vi "Excel Table.vi"(6 "name":string, 8 "error in (no error)":errorcluster, 9 "table":string[][](table), 10 "start (0, 0)":cluster{"row":i32, "column":i32}, 11 "report in":refnum<class "NI_report.lvclass">) -> (0 "error out":errorcluster, 3 "report out":refnum<class "NI_report.lvclass">)   [LabVIEW 2020, in "varilib.lvlib"]
doc: "Inserts a table into a Microsoft Excel report. Do not change the format of cells."
uses:
  varilib.lvlib
  <vilib>/addons/_office/NI_ReportGenerationToolkit.lvlib
  <vilib>/Utility/NIReport.llb/Excel/NI_Excel.lvclass
  <vilib>/Utility/NIReport.llb/NI_report.lvclass
panel:
  in  "column width (1)":dbl=-1.0 format="%0.2f"
  in  "measurement system":u16(ring) caption="measurement system\nfor column width (US)" items=["US", "Metric"]
  out "Row":i32
  out "Column":i32
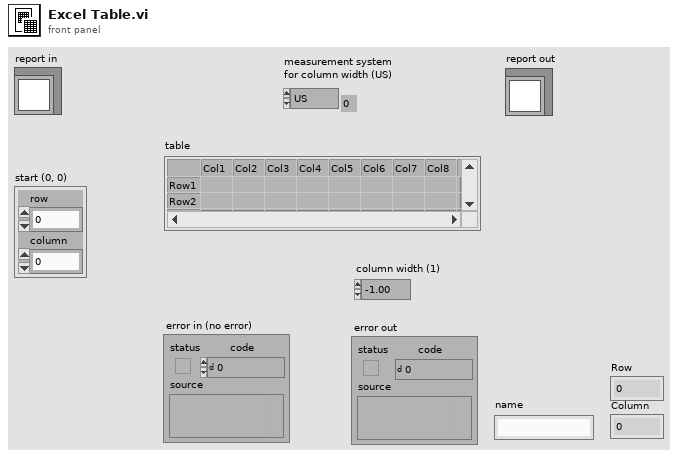
[diagram p1: front panel]
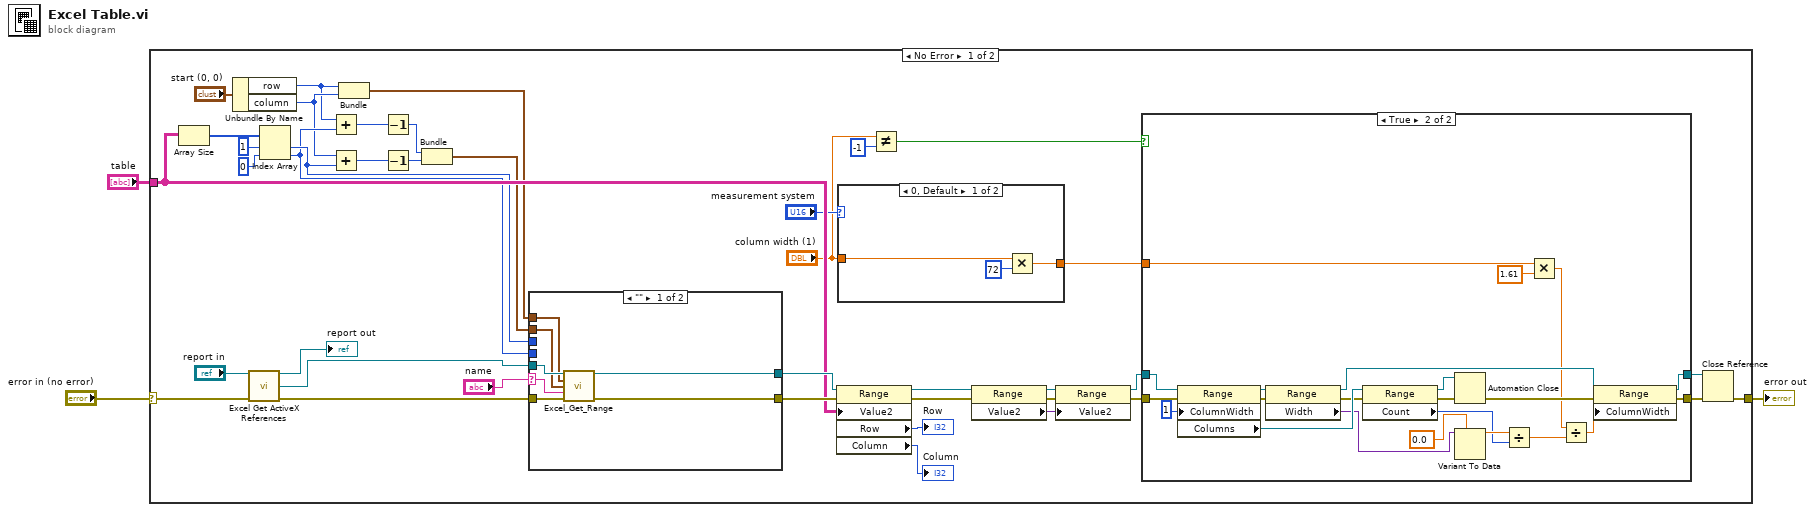
[diagram p0: block diagram]
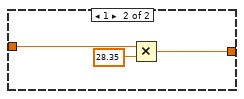
[diagram p2: hidden frame]
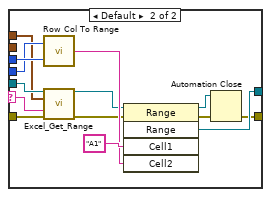
[diagram p4: hidden frame]
diagram:
  n1 = case shown="No Error" "error in (no error)" {
    selector: "error in (no error)" -> [w21 w95]
    tunnel: "table" -> [w39 _]
    tunnel: [w35 w95] -> w2
    frame No Error {
      n2 = Array Size(array=w39) -> (size(s)=w42:i32[])
      n3 = Unbundle By Name("start (0, 0)") -> ("row"=w4:i32, "column"=w5:i32)
      n4 = call <vilib>:"Excel Get ActiveX References.vi"("report in"="report in", "error in (no error)"=w21) -> ("report out"=→"report out":refnum<class "NI_report.lvclass">, "Excel._Worksheet"=w17:refnum<k7>, "error out"=w20:errorcluster)  [unwired: 7 in, 4 out]
      n5 = Index Array(array=w42, index #1=1, index #2=0) -> (element #1=w38:i32, element #2=w23:i32)
      n6 = Add(x=w4, y=w23) -> (x+y=w29:i32)
      n7 = Add(x=w5, y=w38) -> (x+y=w28:i32)
      n8 = Bundle("row"=w4, "column"=w5) -> (w30:cluster{"row":i32, "column":i32})  [unwired: 1 out]
      n9 = Decrement(x=w29) -> (x-1=w26:i32)
      n10 = Decrement(x=w28) -> (x-1=w25:i32)
      n11 = Bundle(w26, w25) -> (w27:cluster{i32, i32})  [unwired: 1 out]
      n12 = case shown="\"\"" "name" {
        selector: "name" -> [w74 w82]
        tunnel: [w80 w94] -> w41
        tunnel: [w79 w88] -> w40
        tunnel: w17 -> [w78 w85]
        tunnel: w20 -> [w77 w84]
        tunnel: w23 -> [_ w90]
        tunnel: w38 -> [_ w91]
        tunnel: w30 -> [w76 w83]
        tunnel: w27 -> [w75 _]
        frame "" {
          n13 = call <vilib>:"Excel_Get_Range.vi"("Excel._Worksheet"=w78, "start"=w76, "end"=w75, "name"=w74, "error in (no error)"=w77) -> ("Range"=w80:refnum<k7>, "error out"=w79:errorcluster)  [unwired: 1 in, 8 out]
        }
        frame Default {
          n14 = call <vilib>:"Row Col To Range.vi"("Column"=w91, "Row"=w90) -> ("Output String"=w92:string)
          n15 = call <vilib>:"Excel_Get_Range.vi"("Excel._Worksheet"=w85, "start"=w83, "name"=w82, "error in (no error)"=w84) -> ("Range"=w81:refnum<k7>, "error out"=w86:errorcluster)  [unwired: 1 in, 9 out]
          n16 = invoke class="Range" method="Range"(reference=w81, error in=w86, "Cell1"="A1", "Cell2"=w92) -> (reference out=w87:refnum<k7>, error out=w89:errorcluster, "Range"=w94:refnum<k7>)  [unwired: 1 in, 2 out]
          n17 = Automation Close(3:w89, 5:w87) -> (0:w88:errorcluster)
        }
      }
      n18 = property class="Range"(reference=w41, error in=w40, "Value2"=w39) -> (reference out=w32:refnum<k7>, error out=w31:errorcluster, "Row"=→"Row":i32, "Column"=→"Column":i32)
      n19 = case shown="0, Default" "measurement system" {
        tunnel: "column width (1)" -> [w46 w48]
        tunnel: [w45 w47] -> w13
        frame 0, Default {
          n20 = Multiply(x=w46, y=72) -> (x*y=w45:dbl)
        }
        frame 1 {
          n21 = Multiply(x=w48, y=28.35) -> (x*y=w47:dbl)
        }
      }
      n22 = Not Equal?(x="column width (1)", y=-1) -> (x != y?=w15:bool)
      n23 = property class="Range"(reference=w32, error in=w31) -> (reference out=w11:refnum<k7>, error out=w10:errorcluster, "Value2"=w7:variant)
      n24 = property class="Range"(reference=w11, error in=w10, "Value2"=w7) -> (reference out=w9:refnum<k7>, error out=w8:errorcluster)
      n25 = case shown="True" w15 {
        tunnel: w9 -> [w51 w73]
        tunnel: w8 -> [w50 w72]
        tunnel: [w50 w70] -> w36
        tunnel: [w51 w71] -> w37
        tunnel: w13 -> [_ w52]
        frame False {
        }
        frame True {
          n26 = property class="Range"(reference=w73, error in=w72, "ColumnWidth"=1) -> (reference out=w59:refnum<k7>, error out=w57:errorcluster, "Columns"=w68:refnum<k7>)
          n27 = property class="Range"(reference=w59, error in=w57) -> (reference out=w58:refnum<k7>, error out=w56:errorcluster, "Width"=w55:variant)
          n28 = property class="Range"(reference=w68, error in=w56) -> (reference out=w64:refnum<k7>, error out=w63:errorcluster, "Count"=w66:i32)
          n29 = Automation Close(3:w63, 5:w64) -> (0:w62:errorcluster)
          n30 = Variant To Data(type=0.0, Variant=w55) -> (data=w67:dbl)  [unwired: 1 in, 1 out]
          n31 = Divide(x=w67, y=w66) -> (x/y=w65:dbl)
          n32 = Multiply(x=w52, y=1.61) -> (x*y=w54:dbl)
          n33 = Divide(x=w54, y=w65) -> (x/y=w61:dbl)
          n34 = property class="Range"(reference=w58, error in=w62, "ColumnWidth"=w61) -> (reference out=w71:refnum<k7>, error out=w70:errorcluster)
        }
      }
      n35 = Close Reference(reference=w37, error in (no error)=w36) -> (error out=w35:errorcluster)
    }
    frame Error {
    }
  }
  "error out" <- w2
